vi "Restore data.vi"(1 "Offset down":sgl format="%.2f", 2 "Offset up":sgl format="%.2f", 3 "Scaled data":sgl[](array[numeric]) format="%.2f") -> (0 "Restored data":sgl[](array[numeric]) format="%.2f")   [LabVIEW 2010]
doc: "This VI scales the data from any range (also negative) into linear range in such a way that minimum input = 0.05 and maximum input = 0.95."
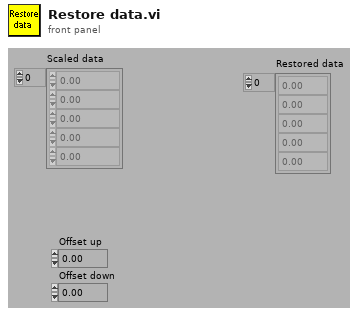
[diagram p1: front panel]
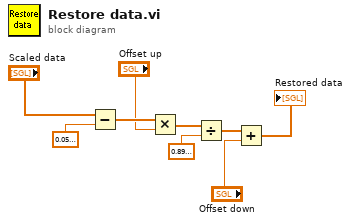
[diagram p0: block diagram]
diagram:
  n1 = Subtract(x="Scaled data", y=sgl 0.05) -> (x-y=w8:sgl[])
  n2 = Multiply(x=w8, y="Offset up") -> (x*y=w6:sgl[])
  n3 = Divide(x=w6, y=sgl 0.9 ("x")) -> (x/y=w4:sgl[])
  n4 = Add(x=w4, y="Offset down") -> (x+y=→"Restored data":sgl[])
